vi "Functional Test.vi"() -> ()   [LabVIEW 2018]
uses:
  api/Failure Information.ctl
  api/Log Record.ctl
  api/logger_class/Internal Log Levels.ctl
  3ae5ef6d-8e83-4c37-89d5-c4af1027e008.vi
  d7f581ef-27d1-4084-8bbe-9e7418d10964.vi
  d7f581ef-27d1-4084-8bbe-9e7418d10964.vi/a153a250-4fb8-4a99-bb5b-6ccb57f1f631.vi
  d7f581ef-27d1-4084-8bbe-9e7418d10964.vi/a153a250-4fb8-4a99-bb5b-6ccb57f1f631.vi/28727e37-b0d9-407c-a479-ab0b7779cd69.vi
  api/configuration/formatters/format_string_formatter/Format String.lvclass
  C:/Users/Colin/Documents/software_projects/glog/src/api/extension/formatter_interface/Formatter.lvclass
  api/configuration/handlers/string_handler/String Handler.lvclass
  C:/Users/Colin/Documents/software_projects/glog/src/api/extension/formatting_handler_interface/Formatting Handler.lvclass
  registry/Log.vi
  api/GLog.lvlib
panel:
  out "failures info":T1[](array[typedef]) {"Log Record"."timestamp" format="%<%x %.3X>T"}
  out "error out":errorcluster
  in  "multi-line w/auto-scroll":string
  in  "single line":string
  in  "multi-line":string
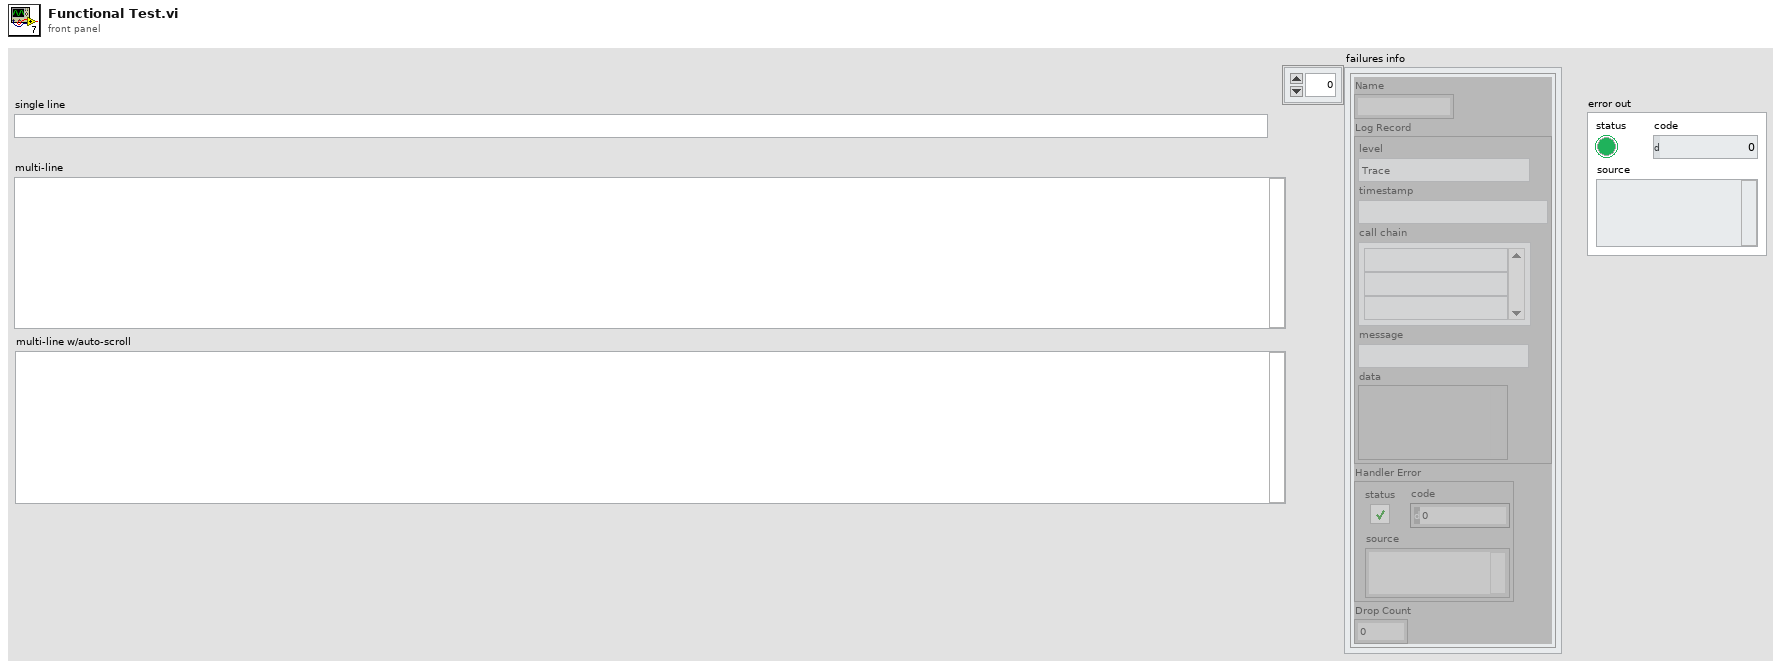
[diagram p1: front panel]
types:
  T1 = typedef "GLog.lvlib/Failure Information.ctl" = cluster{"Name":string, "Log Record":T2, "Handler Error":errorcluster, "Drop Count":u32}
  T2 = typedef "GLog.lvlib/Log Record.ctl" = cluster{"level":T3, "timestamp":timestamp, "call chain":string[], "message":string, "data":variant}
  T3 = typedef "GLog.lvlib/Internal Log Levels.ctl" = enum16{"Trace", "Debug", "Info", "Warning", "Error", "Critical", "Internal"}
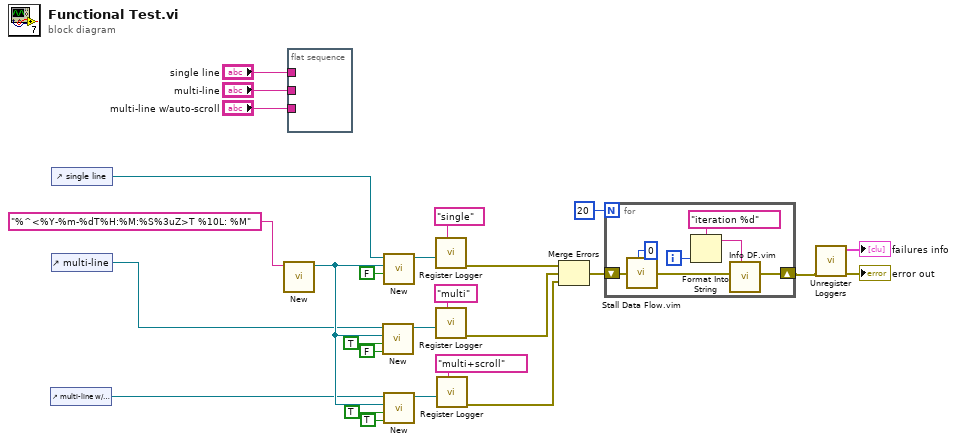
[diagram p0: block diagram]
diagram:
  n1 = control-ref of="multi-line w/auto-scroll"() -> (w19:refnum<vi>)
  n2 = control-ref of="single line"() -> (w21:refnum<vi>)
  n3 = control-ref of="multi-line"() -> (w20:refnum<vi>)
  n4 = call "New.vi"("format string (\"%T | %L | %M\")"="%^<%Y-%m-%dT%H:%M:%S%3uZ>T %10L: %M" ("format string")) -> ("new f-string formatter"=w22:refnum<class "Format String.lvclass">)  [unwired: 10 in]
  n5 = flat-sequence {
    tunnel: "single line" -> [_]
    tunnel: "multi-line" -> [_]
    tunnel: "multi-line w/auto-scroll" -> [_]
    frame #0 {
    }
  }
  n6 = call "New.vi"("auto-scroll? (T)"=FALSE, "multi-line? (T)"=TRUE, "formatter (format string)"=w22, "string control"=w20) -> ("new string handler"=w16:refnum<class "String Handler.lvclass">)  [unwired: 7 in]
  n7 = call "New.vi"("multi-line? (T)"=FALSE, "formatter (format string)"=w22, "string control"=w21) -> ("new string handler"=w18:refnum<class "String Handler.lvclass">)  [unwired: 8 in]
  n8 = call "New.vi"("auto-scroll? (T)"=TRUE, "multi-line? (T)"=TRUE, "formatter (format string)"=w22, "string control"=w19) -> ("new string handler"=w13:refnum<class "String Handler.lvclass">)  [unwired: 7 in]
  n9 = call "Register Logger.vi"("name (\"Default\")"="single" ("name (\"Default\")"), "log handler (file handler)"=w18) -> ("error out"=w12:errorcluster)  [unwired: 9 in]
  n10 = call "Register Logger.vi"("name (\"Default\")"="multi" ("name (\"Default\")"), "log handler (file handler)"=w16) -> ("error out"=w11:errorcluster)  [unwired: 9 in]
  n11 = call "Register Logger.vi"("name (\"Default\")"="multi+scroll" ("name (\"Default\")"), "log handler (file handler)"=w13) -> ("error out"=w10:errorcluster)  [unwired: 9 in]
  n12 = Merge Errors(w12, w11, w10) -> (w9:errorcluster)
  n13 = for {
    N: 20 -> [_]
    shift-right: [w29] -> w2
    shift-left: w9 -> [w33]
    i -> [w32]
    n14 = call "Stall Data Flow.vim"("value in"=w33, "milliseconds to wait"=u32 0) -> ("value out"=w28:errorcluster)  [unwired: 1 out]
    n15 = Format Into String(format string="iteration %d", w32) -> (resulting string=w30:string)  [unwired: 2 in, 1 out]
    n16 = call "Info DF.vim"("message"=w30, "dataflow in"=w28) -> ("dataflow out"=w29:errorcluster)  [unwired: 9 in]
  }
  n17 = call "Unregister Loggers.vi"("error in (no error)"=w2) -> ("error out"=→"error out":errorcluster, "failures info"=→"failures info":T1[])  [unwired: 9 in]
